vi "Apply Topology Mode.vi"(8 "error in":errorcluster, 11 "SwitchMatrix in":refnum<class "SwitchMatrix.lvclass">) -> (0 "error out":errorcluster, 3 "SwitchMatrix out":refnum<class "SwitchMatrix.lvclass">)   [LabVIEW 2019, in "SwitchMatrix.lvlib" / "SwitchMatrix.lvclass"]
uses:
  Library/SwitchMatrix.lvclass
  Custom Controls/Topology_Mode.ctl
  Library/SwitchMatrix.lvclass/SwitchMatrix.ctl
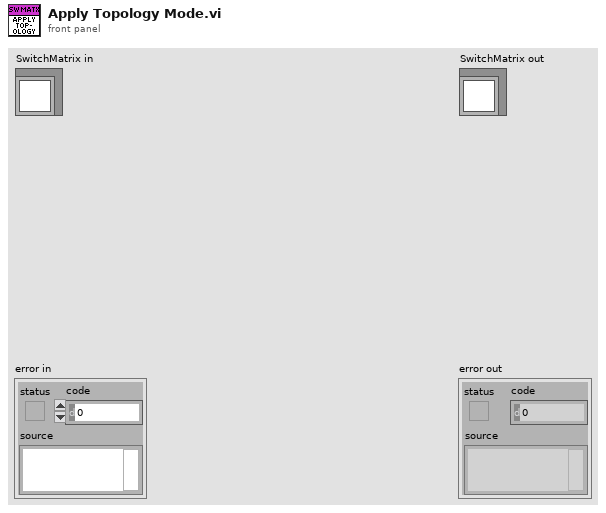
[diagram p1: front panel]
types:
  T1 = typedef "SwitchMatrix.lvlib/SwitchMatrix.lvclass/Topology_Mode.ctl" = enum16{"Single", "Dual", "Quad", "Octal", "Sixteen"}
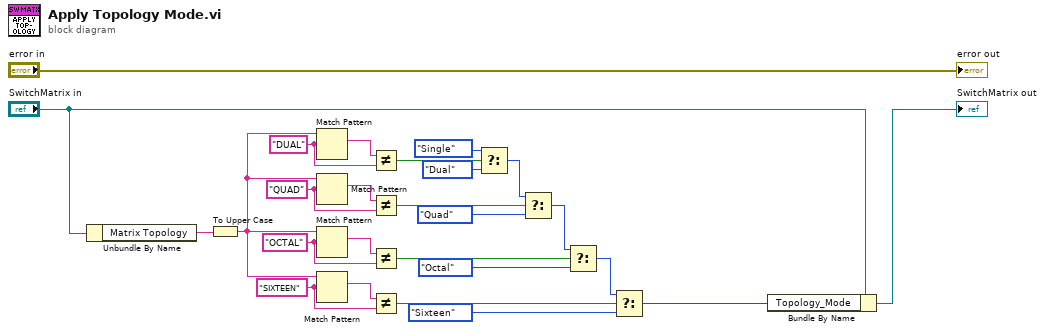
[diagram p0: block diagram]
diagram:
  w12 = "SIXTEEN" ("regular expression")
  w11 = "OCTAL" ("regular expression")
  w18 = "QUAD" ("regular expression")
  w21 = "DUAL" ("regular expression")
  n1 = Unbundle By Name("SwitchMatrix in") -> ("Matrix Topology"=w1:string)
  n2 = To Upper Case(1:w1) -> (0:w2:string)
  n3 = Match Pattern(string=w2, regular expression=w21) -> (match substring=w22:string)  [unwired: 1 in, 3 out]
  n4 = Match Pattern(string=w2, regular expression=w18) -> (match substring=w17:string)  [unwired: 1 in, 3 out]
  n5 = Match Pattern(string=w2, regular expression=w11) -> (match substring=w10:string)  [unwired: 1 in, 3 out]
  n6 = Match Pattern(string=w2, regular expression=w12) -> (match substring=w13:string)  [unwired: 1 in, 3 out]
  n7 = Not Equal?(x=w22, y=w21) -> (x != y?=w20:bool)
  n8 = Not Equal?(x=w17, y=w18) -> (x != y?=w16:bool)
  n9 = Not Equal?(x=w10, y=w11) -> (x != y?=w9:bool)
  n10 = Not Equal?(x=w13, y=w12) -> (x != y?=w8:bool)
  n11 = Select(t=Topology_Mode."Single" ("Topology_Mode"), s=w20, f=Topology_Mode."Dual" ("Topology_Mode")) -> (s? t:f=w19:T1)
  n12 = Select(t=w19, s=w16, f=Topology_Mode."Quad" ("Topology_Mode")) -> (s? t:f=w15:T1)
  n13 = Select(t=w15, s=w9, f=Topology_Mode."Octal" ("Topology_Mode")) -> (s? t:f=w14:T1)
  n14 = Select(t=w14, s=w8, f=Topology_Mode."Sixteen" ("Topology_Mode")) -> (s? t:f=w3:T1)
  n15 = Bundle By Name(cluster="SwitchMatrix in", "Topology_Mode"=w3) -> (→"SwitchMatrix out":refnum<class "SwitchMatrix.lvclass">)
  "error out" <- "error in"
